vi "pulse input show for photo.vi"() -> ()   [LabVIEW 2023]
uses:
  <vilib>/DAQmx/read.llb/DAQmx Read (Analog 1D Wfm NChan NSamp).vi
  <vilib>/DAQmx/write.llb/DAQmx Write (Analog 1D Wfm NChan NSamp).vi
  <vilib>/DAQmx/create/channels.llb/DAQmx Create Channel (AI-Voltage-Basic).vi
  <vilib>/DAQmx/configure/timing.llb/DAQmx Timing (Sample Clock).vi
  <vilib>/DAQmx/create/channels.llb/DAQmx Create Channel (AO-Voltage-Basic).vi
  <vilib>/DAQmx/miscellaneous.llb/DAQmx Fill In Error Info.vi
panel:
  out "Duty Cycle 4":dbl
  out "Period 4":dbl
  out "Frequency 4":dbl
  out "Duty Cycle 3":dbl
  out "Period 3":dbl
  out "Frequency 3":dbl
  out "Waveform Graph 2":dynamicdata(graph)
  in  "physical channels 2":tag
  in  "physical channels":tag
  out "Duty Cycle 2":dbl
  out "Period 2":dbl
  out "Frequency 2":dbl
  out "Duty Cycle":dbl
  out "Period":dbl
  out "Frequency":dbl
  out "Waveform Graph":dynamicdata(graph)
  in  "stop":bool
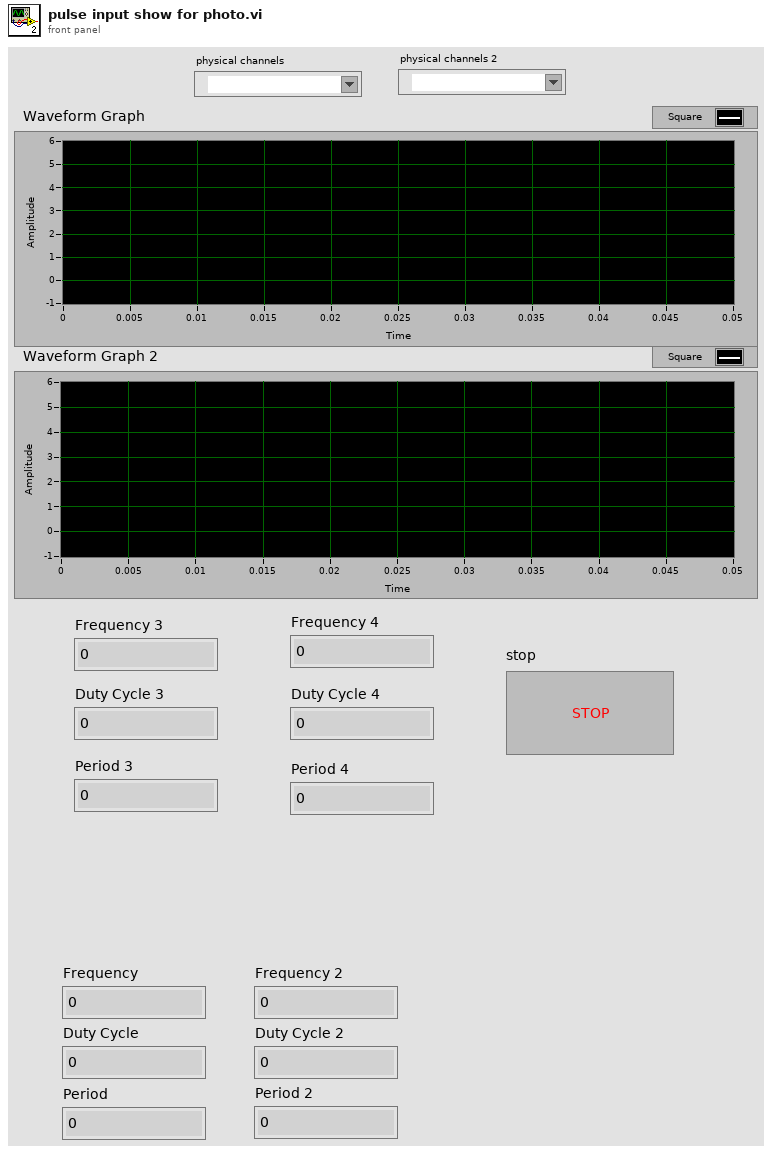
[diagram p1: front panel]
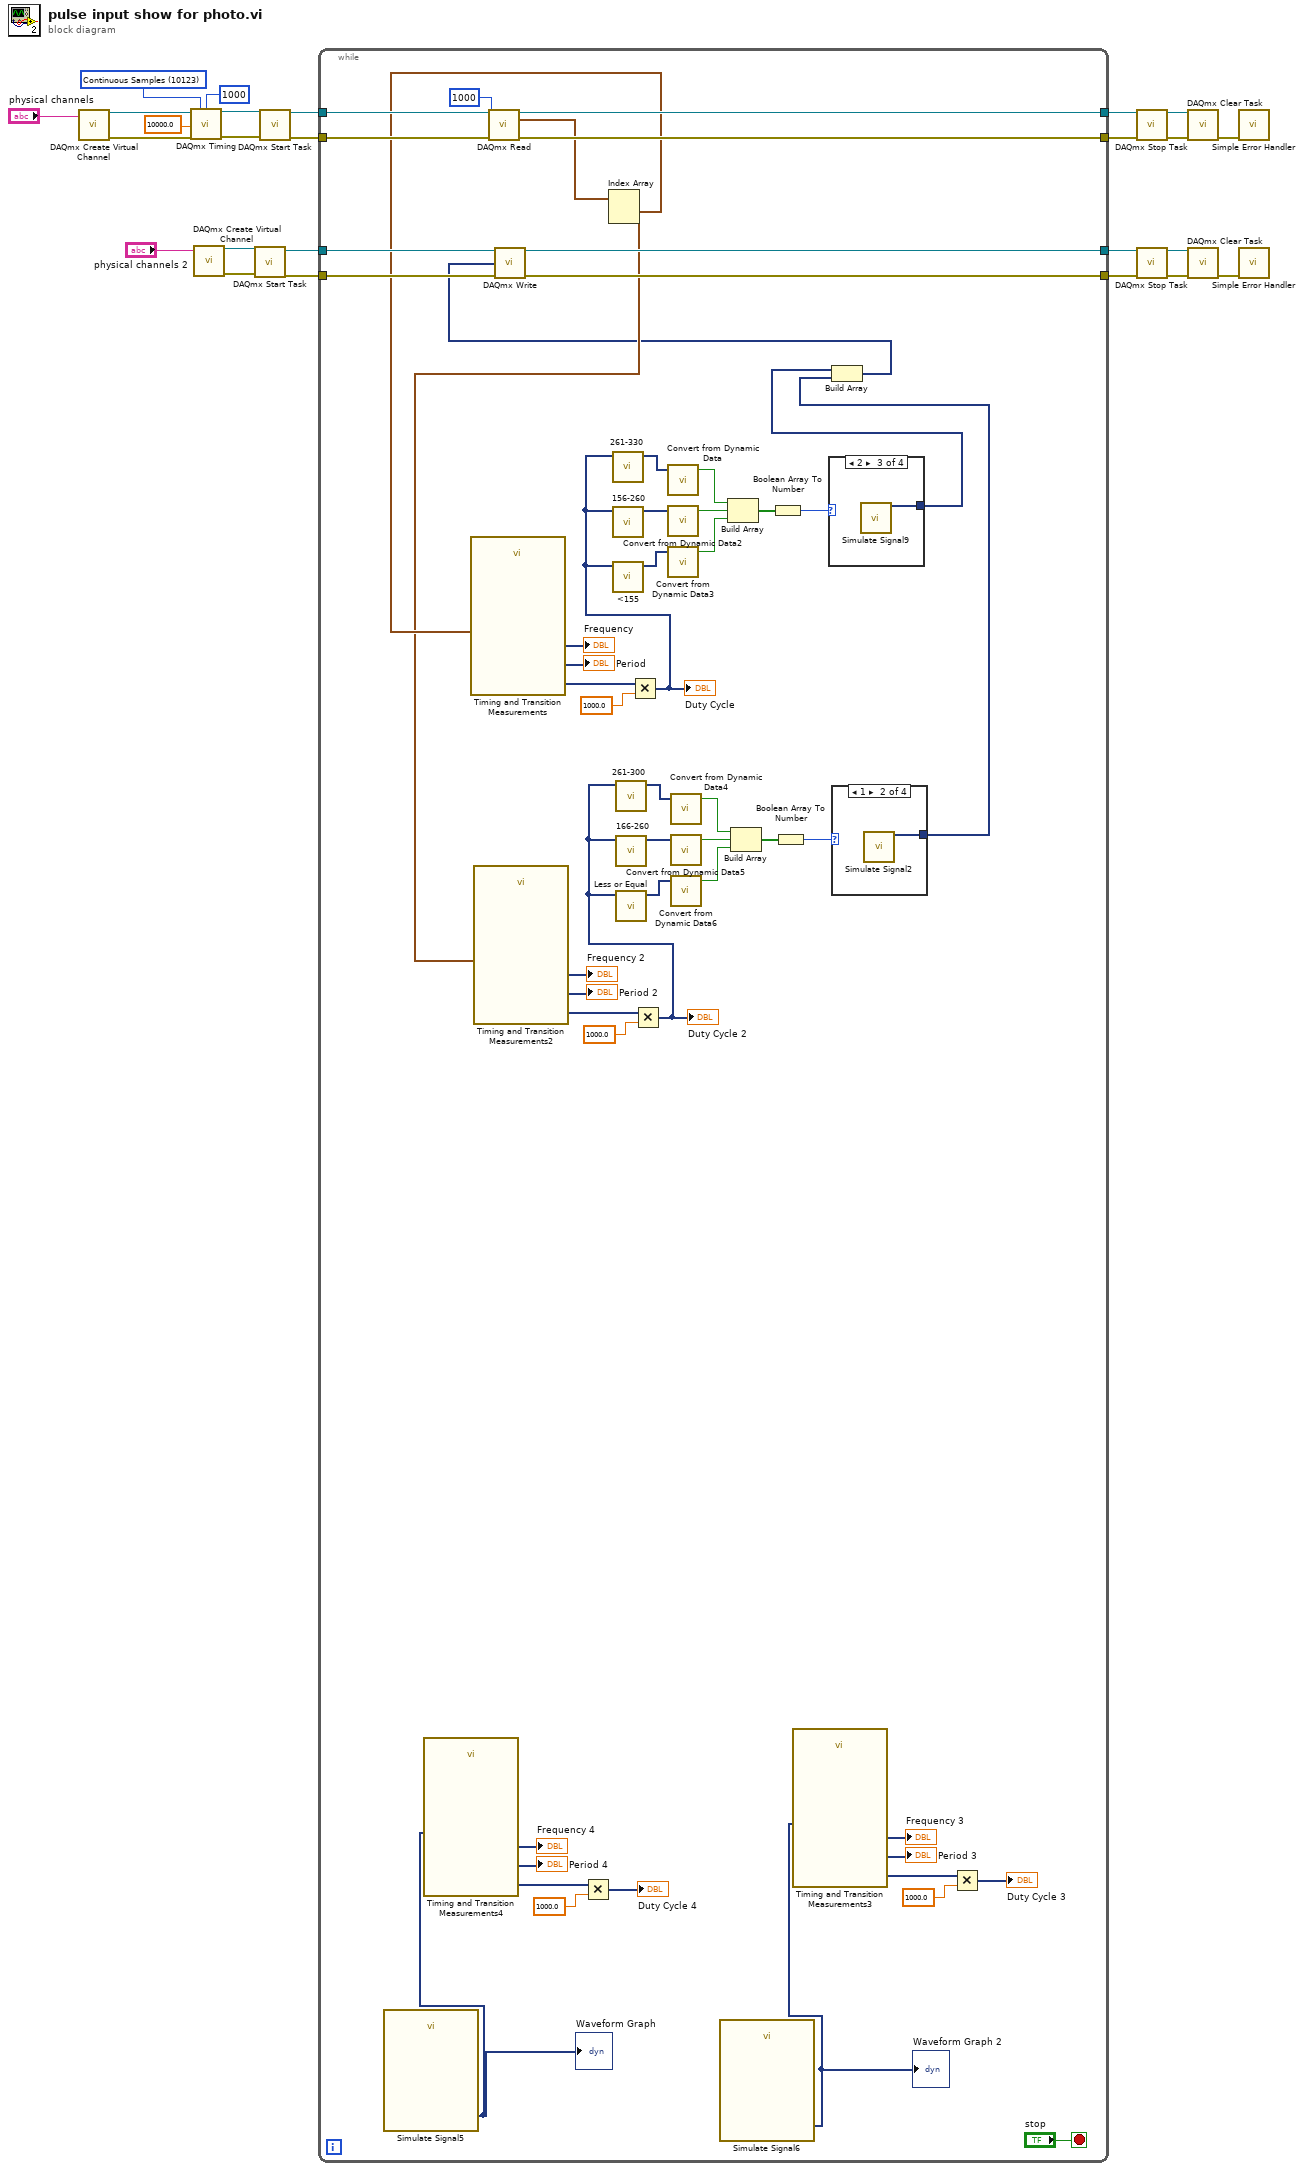
[diagram p0: block diagram]
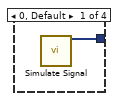
[diagram p2: hidden frame]
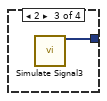
[diagram p3: hidden frame]
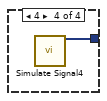
[diagram p4: hidden frame]
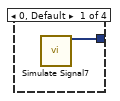
[diagram p5: hidden frame]
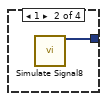
[diagram p6: hidden frame]
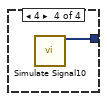
[diagram p7: hidden frame]
diagram:
  w17 = 10123 items=["Finite Samples"=10178, "Continuous Samples"=10123, "Hardware Timed Single Point"=12522] ("sample mode")
  n1 = call-poly <vilib>:"DAQmx Create Virtual Channel.vi"("physical channels"="physical channels") -> ("task out"=w22:refnum<k21>, "error out"=w21:errorcluster)  [unwired: 13 in]
  n2 = call-poly <vilib>:"DAQmx Timing.vi"("task/channels in"=w22, "sample mode"=w17, "samples per channel"=1000, "rate"=10000.0, "error in"=w21) -> ("task out"=w19:refnum<k21>, "error out"=w20:errorcluster)  [unwired: 9 in]
  n3 = call-poly <vilib>:"DAQmx Create Virtual Channel.vi"("physical channels"="physical channels 2") -> ("task out"=w15:refnum<k21>, "error out"=w14:errorcluster)  [unwired: 13 in]
  n4 = call <vilib>:"DAQmx Start Task.vi"("task/channels in"=w15, "error in"=w14) -> ("task out"=w10:refnum<k21>, "error out"=w8:errorcluster)  [unwired: 12 in]
  n5 = call <vilib>:"DAQmx Start Task.vi"("task/channels in"=w19, "error in"=w20) -> ("task out"=w6:refnum<k21>, "error out"=w5:errorcluster)  [unwired: 12 in]
  n6 = while {
    tunnel: w10 -> [w52]
    tunnel: [w51] -> w9
    tunnel: w8 -> [w50]
    tunnel: [w49] -> w7
    tunnel: w6 -> [w47]
    tunnel: [w45] -> w4
    tunnel: w5 -> [w46]
    tunnel: [w44] -> w3
    stop <- "stop" stop-if-true
    n7 = call "Simulate Signal5"() -> ("Square"=w26:dynamicdata)  [unwired: 14 in, 1 out]
    "Waveform Graph" <- w26
    n8 = call "Timing and Transition Measurements4"("Signals"=w26) -> ("Frequency"=→"Frequency 4":dynamicdata, "Period"=→"Period 4":dynamicdata, "Duty Cycle"=w30:dynamicdata)  [unwired: 7 in, 1 out]
    n9 = call-poly <vilib>:"DAQmx Read.vi"("task/channels in"=w47, "number of samples per channel"=1000, "error in"=w46) -> ("task out"=w45:refnum<k21>, "data"=w43:waveform(dbl)[], "error out"=w44:errorcluster)  [unwired: 10 in]
    n10 = Multiply(x=w30, y=1000.0) -> (x*y=→"Duty Cycle 4":dynamicdata)
    n11 = Index Array(array=w43) -> (element #1=w42:waveform(dbl), element #2=w41:waveform(dbl))  [unwired: 2 in]
    n12 = call "Timing and Transition Measurements"("Signals"=w42) -> ("Frequency"=→"Frequency":dynamicdata, "Period"=→"Period":dynamicdata, "Duty Cycle"=w76:dynamicdata)  [unwired: 7 in, 1 out]
    n13 = call "Timing and Transition Measurements2"("Signals"=w41) -> ("Frequency"=→"Frequency 2":dynamicdata, "Period"=→"Period 2":dynamicdata, "Duty Cycle"=w63:dynamicdata)  [unwired: 7 in, 1 out]
    n14 = Multiply(x=w76, y=1000.0) -> (x*y=w74:dynamicdata)
    "Duty Cycle" <- w74
    n15 = call "261-330"("Operand 1"=w74) -> ("Result"=w73:dynamicdata)  [unwired: 9 in, 1 out]
    n16 = call "156-260"("Operand 1"=w74) -> ("Result"=w72:dynamicdata)  [unwired: 9 in, 1 out]
    n17 = call "<155"("Operand 1"=w74) -> ("Result"=w71:dynamicdata)  [unwired: 9 in, 1 out]
    n18 = Multiply(x=w63, y=1000.0) -> (x*y=w61:dynamicdata)
    "Duty Cycle 2" <- w61
    n19 = call "261-300"("Operand 1"=w61) -> ("Result"=w60:dynamicdata)  [unwired: 9 in, 1 out]
    n20 = call "166-260"("Operand 1"=w61) -> ("Result"=w59:dynamicdata)  [unwired: 9 in, 1 out]
    n21 = call "Less or Equal"("Operand 1"=w61) -> ("Result"=w58:dynamicdata)  [unwired: 9 in, 1 out]
    n22 = call "Convert from Dynamic Data"("Dynamic Data Type"=w73) -> ("Scalar"=w69:bool)  [unwired: 3 in]
    n23 = call "Convert from Dynamic Data2"("Dynamic Data Type"=w72) -> ("Scalar"=w70:bool)  [unwired: 3 in]
    n24 = call "Convert from Dynamic Data3"("Dynamic Data Type"=w71) -> ("Scalar"=w68:bool)  [unwired: 3 in]
    n25 = call "Convert from Dynamic Data4"("Dynamic Data Type"=w60) -> ("Scalar"=w56:bool)  [unwired: 3 in]
    n26 = call "Convert from Dynamic Data5"("Dynamic Data Type"=w59) -> ("Scalar"=w57:bool)  [unwired: 3 in]
    n27 = call "Convert from Dynamic Data6"("Dynamic Data Type"=w58) -> ("Scalar"=w55:bool)  [unwired: 3 in]
    n28 = call "Simulate Signal6"() -> ("Square"=w27:dynamicdata)  [unwired: 14 in, 1 out]
    "Waveform Graph 2" <- w27
    n29 = Build Array(w69, w70, w68) -> (w67:bool[])
    n30 = Build Array(w56, w57, w55) -> (w54:bool[])
    n31 = Boolean Array To Number(Boolean array=w67) -> (number=w66:u32)
    n32 = Boolean Array To Number(Boolean array=w54) -> (number=w53:u32)
    n33 = call "Timing and Transition Measurements3"("Signals"=w27) -> ("Frequency"=→"Frequency 3":dynamicdata, "Period"=→"Period 3":dynamicdata, "Duty Cycle"=w35:dynamicdata)  [unwired: 7 in, 1 out]
    n34 = case shown="2" w66 {
      tunnel: [w84 w85 w86 w87] -> w40
      frame 0, Default {
        n35 = call "Simulate Signal7"() -> ("DC"=w84:dynamicdata)  [unwired: 14 in, 1 out]
      }
      frame 1 {
        n36 = call "Simulate Signal8"() -> ("Square"=w85:dynamicdata)  [unwired: 14 in, 1 out]
      }
      frame 2 {
        n37 = call "Simulate Signal9"() -> ("Square"=w86:dynamicdata)  [unwired: 14 in, 1 out]
      }
      frame 4 {
        n38 = call "Simulate Signal10"() -> ("DC"=w87:dynamicdata)  [unwired: 14 in, 1 out]
      }
    }
    n39 = case shown="1" w53 {
      tunnel: [w80 w81 w82 w83] -> w39
      frame 0, Default {
        n40 = call "Simulate Signal"() -> ("DC"=w80:dynamicdata)  [unwired: 14 in, 1 out]
      }
      frame 1 {
        n41 = call "Simulate Signal2"() -> ("Square"=w81:dynamicdata)  [unwired: 14 in, 1 out]
      }
      frame 2 {
        n42 = call "Simulate Signal3"() -> ("Square"=w82:dynamicdata)  [unwired: 14 in, 1 out]
      }
      frame 4 {
        n43 = call "Simulate Signal4"() -> ("DC"=w83:dynamicdata)  [unwired: 14 in, 1 out]
      }
    }
    n44 = Build Array(w40, w39) -> (w38:dynamicdata[])
    n45 = call-poly <vilib>:"DAQmx Write.vi"("task/channels in"=w52, "data"=w38, "error in"=w50) -> ("task out"=w51:refnum<k21>, "error out"=w49:errorcluster)  [unwired: 10 in, 1 out]
    n46 = Multiply(x=w35, y=1000.0) -> (x*y=→"Duty Cycle 3":dynamicdata)
  }
  n47 = call <vilib>:"DAQmx Stop Task.vi"("task/channels in"=w4, "error in"=w3) -> ("task out"=w25:refnum<k21>, "error out"=w23:errorcluster)  [unwired: 12 in]
  n48 = call <vilib>:"DAQmx Stop Task.vi"("task/channels in"=w9, "error in"=w7) -> ("task out"=w13:refnum<k21>, "error out"=w11:errorcluster)  [unwired: 12 in]
  n49 = call <vilib>:"DAQmx Clear Task.vi"("task in"=w25, "error in"=w23) -> ("error out"=w24:errorcluster)  [unwired: 13 in]
  n50 = call <vilib>:"DAQmx Clear Task.vi"("task in"=w13, "error in"=w11) -> ("error out"=w12:errorcluster)  [unwired: 13 in]
  n51 = call <vilib>:"Simple Error Handler.vi"("error in (no error)"=w24) -> ()  [unwired: 4 in, 5 out]
  n52 = call <vilib>:"Simple Error Handler.vi"("error in (no error)"=w12) -> ()  [unwired: 4 in, 5 out]
